vi "as UINT8.vi"(11 "bytes":u8[](array[numeric]) format="%b") -> (3 "UINT8":u8)   [LabVIEW 2020, in "MessagePack.lvlib" / "MessagePackNumeric.lvclass"]
uses:
  MessagePackNumeric.lvclass
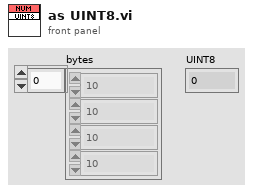
[diagram p1: front panel]
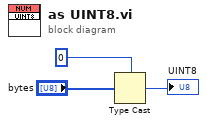
[diagram p0: block diagram]
diagram:
  n1 = Type Cast(type=u8 0 ("INT8"), x="bytes") -> (*(type *) &x=→"UINT8":u8)
